vi "svl_Integration No State.vi"(0 "scaled signal [EU]":waveform(dbl), 1 "reset filters":bool, 2 "length units":i32(ring) items=["no change"=-1, "m"=0, "mm"=2, "microns"=3, "in"=1, "mils"=5], 5 "integration type":T3(ring), 7 "highpass cutoff frequency":dbl format="%.2f", 9 "filter coefficents in":T2 {"highpass filter coefficients"."Forward Coefficients" format="%.2f"; "highpass filter coefficients"."Reverse Coefficients" format="%.2f"; "integration filter coefficients"."alpha" format="%.2f"; "integration filter coefficients"."gamma" format="%.2f"; "integration filter coefficients"."beta" format="%.2f"}, 11 "error in (no error)":errorcluster, 12 "initial filter state":T1 {"initial highpass filter state" format="%.2f"; "initial integration fiter state"."y(n-2) state" format="%.2f"; "initial integration fiter state"."x(n-2) state" format="%.2f"; "initial integration fiter state"."y(n-1) state" format="%.2f"; "initial integration fiter state"."x(n-1) state" format="%.2f"}) -> (4 "scaled signal [EU]":waveform(dbl), 6 "unit label":string, 10 "filter coefficients out":T2 {"highpass filter coefficients"."Forward Coefficients" format="%.2f"; "highpass filter coefficients"."Reverse Coefficients" format="%.2f"; "integration filter coefficients"."alpha" format="%.2f"; "integration filter coefficients"."gamma" format="%.2f"; "integration filter coefficients"."beta" format="%.2f"}, 14 "final filter state":T1 {"initial highpass filter state" format="%.2f"; "initial integration fiter state"."y(n-2) state" format="%.2f"; "initial integration fiter state"."x(n-2) state" format="%.2f"; "initial integration fiter state"."y(n-1) state" format="%.2f"; "initial integration fiter state"."x(n-1) state" format="%.2f"}, 15 "error out":errorcluster)   [LabVIEW 2017, in "SoundVib_Integration.lvlib"]
uses:
  <vilib>/addons/Sound and Vibration/svt_Integration/SoundVib_Integration.lvlib
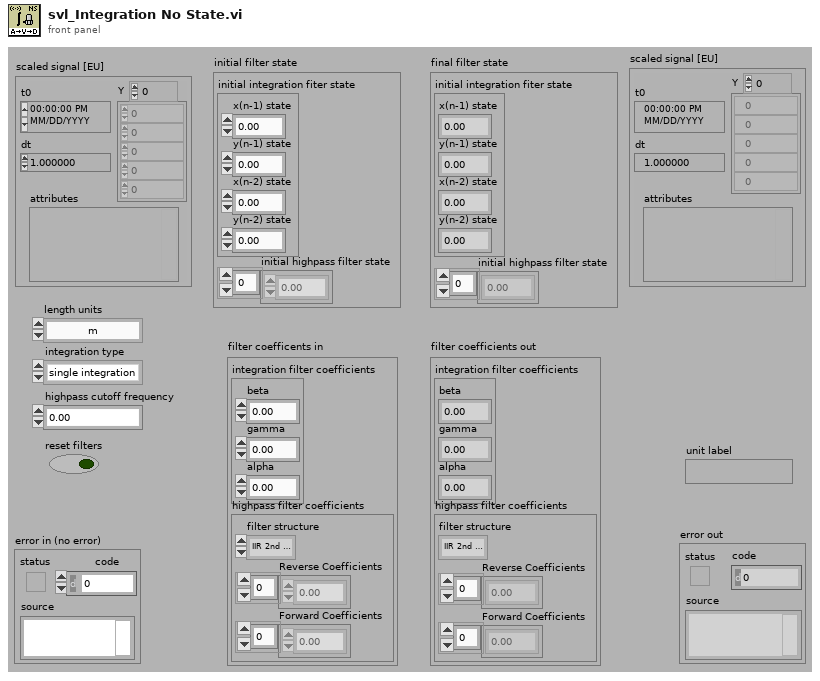
[diagram p1: front panel]
types:
  T1 = cluster{"initial integration fiter state":cluster{"x(n-1) state":dbl, "y(n-1) state":dbl, "x(n-2) state":dbl, "y(n-2) state":dbl}, "initial highpass filter state":dbl[]}
  T2 = cluster{"integration filter coefficients":cluster{"beta":dbl, "gamma":dbl, "alpha":dbl}, "highpass filter coefficients":cluster{"filter structure":enum32{"IIR 2nd Order", "IIR 4th Order"}, "Reverse Coefficients":dbl[], "Forward Coefficients":dbl[]}}
  T3 = enum16{"single integration", "double integration"}
  T4 = cluster{"filter structure":enum32{"IIR 2nd Order", "IIR 4th Order"}, "Reverse Coefficients":dbl[], "Forward Coefficients":dbl[]}
  T5 = cluster{"x(n-1) state":dbl, "y(n-1) state":dbl, "x(n-2) state":dbl, "y(n-2) state":dbl}
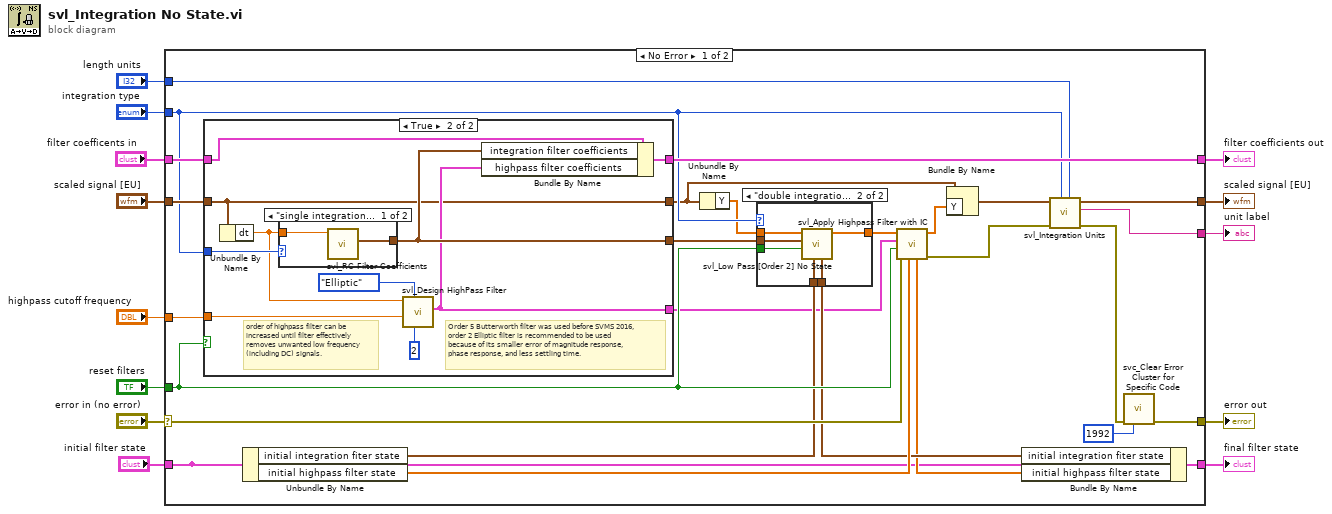
[diagram p0: block diagram]
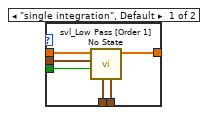
[diagram p2: hidden frame]
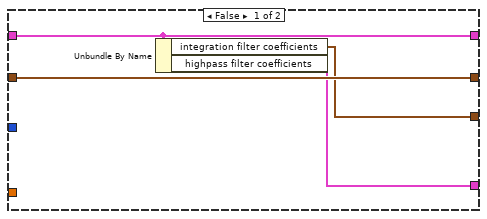
[diagram p3: hidden frame]
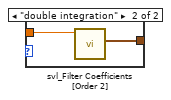
[diagram p4: hidden frame]
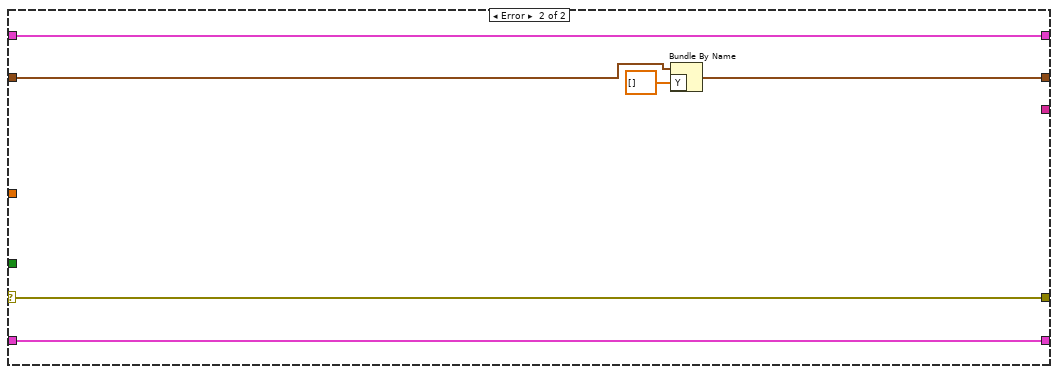
[diagram p5: hidden frame]
diagram:
  n1 = case shown="No Error" "error in (no error)" {
    selector: "error in (no error)" -> [w37 w76]
    tunnel: "reset filters" -> [w38 _]
    tunnel: "highpass cutoff frequency" -> [w39 _]
    tunnel: "scaled signal [EU]" -> [w40 w71]
    tunnel: [w20 w74] -> w7
    tunnel: "integration type" -> [w25 _]
    tunnel: [w22 w76] -> w8
    tunnel: "length units" -> [w24 _]
    tunnel: [w26 _] -> w9
    tunnel: "initial filter state" -> [w23 w73]
    tunnel: "filter coefficents in" -> [w31 w72]
    tunnel: [w32 w73] -> w2
    tunnel: [w28 w72] -> w1
    frame No Error {
      n2 = case shown="True" w38 {
        tunnel: w25 -> [_ w66]
        tunnel: w40 -> [w56 w59]
        tunnel: [w56 w59] -> w16
        tunnel: w39 -> [_ w65]
        tunnel: [w54 w62] -> w30
        tunnel: [w55 w63] -> w29
        tunnel: w31 -> [w53 w60]
        tunnel: [w53 w61] -> w28
        frame False {
          n3 = Unbundle By Name(w53) -> ("integration filter coefficients"=w55:cluster{"beta":dbl, "gamma":dbl, "alpha":dbl}, "highpass filter coefficients"=w54:T4)
        }
        frame True {
          # "Order 5 Butterworth filter was used before SVMS 2016, \norder 2 Elliptic filter is recommended to be used \nbecause of its smaller error of magnitude response, \nphase response, and less settling time."
          # "order of highpass filter can be\nincreased until filter effectively\nremoves unwanted low frequency\n(including DC) signals."
          n4 = Unbundle By Name(w59) -> ("dt"=w58:dbl)
          n5 = case shown="\"single integration\", Default" w66 {
            tunnel: [w68 w70] -> w63
            tunnel: w58 -> [w67 w69]
            frame "single integration", Default {
              n6 = call <vilib>:"svl_RC Filter Coefficients.vi"("dt"=w67) -> ("filter coefficients"=w68:cluster{"beta":dbl, "gamma":dbl, "alpha":dbl})  [unwired: 10 in]
            }
            frame "double integration" {
              n7 = call <vilib>:"svl_Filter Coefficients [Order 2].vi"("dt"=w69) -> ("filter coefficients"=w70:cluster{"beta":dbl, "gamma":dbl, "alpha":dbl})  [unwired: 10 in]
            }
          }
          n8 = call <vilib>:"svl_Design HighPass Filter.vi"("highpass filter order"=2 ("order of filter can be\nincreased until filter\neffectively removes\nunwanted low\nfrequency (including\nDC) signals."), "filter design method"=enum16{"Elliptic", "Butterworth"}."Elliptic", "highpass cutoff frequency"=w65, "dt"=w58) -> ("IIR Filter Cluster"=w62:T4)  [unwired: 6 in, 1 out]
          n9 = Bundle By Name(cluster=w60, "integration filter coefficients"=w63, "highpass filter coefficients"=w62) -> (w61:T2)
        }
      }
      n10 = Unbundle By Name(w23) -> ("initial integration fiter state"=w35:T5, "initial highpass filter state"=w36:dbl[])
      n11 = Unbundle By Name(w16) -> ("Y"=w18:dbl[])
      n12 = case shown="\"double integration\"" w25 {
        tunnel: w18 -> [w46 w52]
        tunnel: [w45 w51] -> w17
        tunnel: w29 -> [w44 w50]
        tunnel: w38 -> [w43 w49]
        tunnel: [w41 w48] -> w34
        tunnel: w35 -> [w42 w47]
        frame "single integration", Default {
          n13 = call <vilib>:"svl_Low Pass [Order 1] No State.vi"("state info in"=w42, "reset"=w43, "filter coefficients"=w44, "Input stream"=w46) -> ("filtered signal"=w45:dbl[], "state info out"=w41:T5)  [unwired: 6 in]
        }
        frame "double integration" {
          n14 = call <vilib>:"svl_Low Pass [Order 2] No State.vi"("state info in"=w47, "reset"=w49, "filter coefficients"=w50, "Input stream"=w52) -> ("filtered signal"=w51:dbl[], "state info out"=w48:T5)  [unwired: 6 in]
        }
      }
      n15 = call <vilib>:"svl_Apply Highpass Filter with IC.vi"("Initial Filter State"=w36, "error in (no error)"=w37, "reset"=w38, "filter coefficients"=w30, "signal [V]"=w17) -> ("error out"=w27:errorcluster, "filtered signal [EU]"=w15:dbl[], "Final Filter State"=w33:dbl[])  [unwired: 4 in]
      n16 = Bundle By Name(cluster=w16, "Y"=w15) -> (w14:waveform(dbl))
      n17 = Bundle By Name(cluster=w23, "initial integration fiter state"=w34, "initial highpass filter state"=w33) -> (w32:T1)
      n18 = call <vilib>:"svl_Integration Units.vi"("desired base units for length"=w24, "integration type"=w25, "error in (no error)"=w27, "scaled signal [EU]"=w14) -> ("error out"=w19:errorcluster, "unit label"=w26:string, "scaled signal out"=w20:waveform(dbl))  [unwired: 5 in]
      n19 = call <vilib>:"svc_Clear Error Cluster for Specific Code.vi"("error in (no error)"=w19, "code"=1992) -> ("error out"=w22:errorcluster)  [unwired: 12 in, 1 out]
    }
    frame Error {
      n20 = Bundle By Name(cluster=w71, "Y"=dbl[] []) -> (w74:waveform(dbl))
    }
  }
  "unit label" <- w9
  "error out" <- w8
  "scaled signal [EU]" <- w7
  "filter coefficients out" <- w1
  "final filter state" <- w2
